vi "start.vi"(8 "error in (no error)":errorcluster, 11 "NetworkWinX32 in":refnum<class "NetworkWinX32.lvclass">) -> (0 "error out":errorcluster, 3 "NetworkWinX32 out":refnum<class "NetworkWinX32.lvclass">)   [LabVIEW 2011, in "Hardware.lvlib" / "HWControllers.lvlib" / "NetworkWinX32.lvclass"]
uses:
  NetworkWinX32.lvclass
  NetworkWinX32.lvclass/NetworkWinX32.ctl
  Channels/Camera/WinX32_SA/WinX32Camera.lvclass
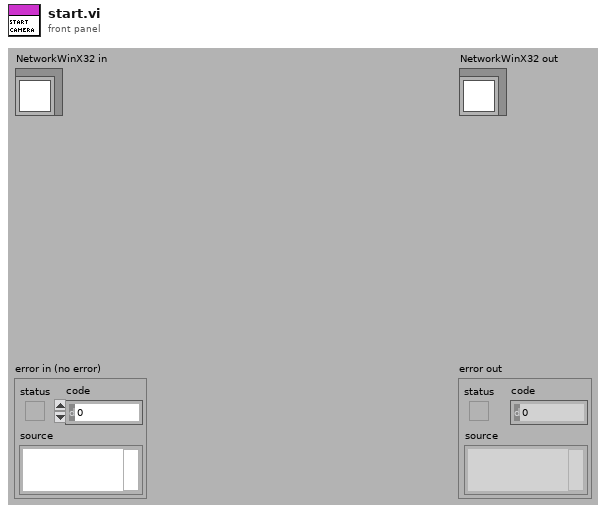
[diagram p1: front panel]
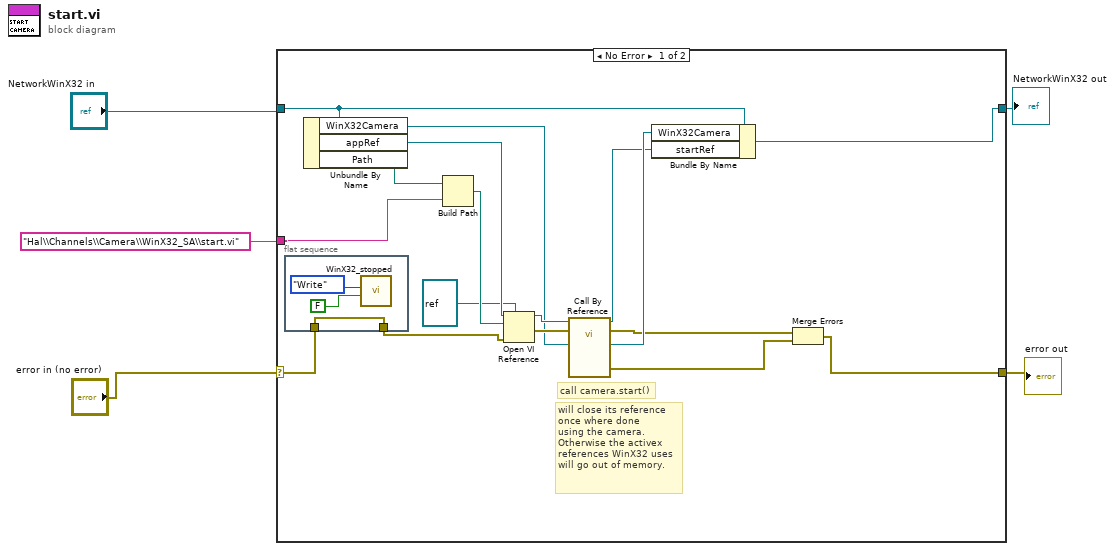
[diagram p0: block diagram]
diagram:
  n1 = case shown="No Error" "error in (no error)" {
    selector: "error in (no error)" -> [w9 w27]
    tunnel: [w11 w27] -> w2
    tunnel: [w10 w26] -> w3
    tunnel: "NetworkWinX32 in" -> [w14 w26]
    tunnel: "Hal\\Channels\\Camera\\WinX32_SA\\start.vi" ("viPath") -> [w21 _]
    frame No Error {
      # "will close its reference\nonce where done\nusing the camera.\nOtherwise the activex\nreferences WinX32 uses\nwill go out of memory."
      # "call camera.start()"
      n2 = flat-sequence {
        tunnel: w9 -> [w25]
        tunnel: [w25] -> w8
        frame #0 {
          n3 = call "WinX32_stopped.vi"("stop"=FALSE, "Action"=enum16{"Write", "Read"}."Write") -> ()  [unwired: 9 in, 1 out]
        }
      }
      n4 = Unbundle By Name(w14) -> ("WinX32Camera"=w15:refnum<class "WinX32Camera.lvclass">, "appRef"=w19:refnum<vi>, "Path"=w20:path)
      n5 = Build Path(base path=w20, name or relative path=w21) -> (appended path=w22:path)
      n6 = Open VI Reference(type specifier VI Refnum (for type only)=refnum<vi> refnum, application reference (local)=w19, vi path=w22, error in (no error)=w8) -> (vi reference=w17:refnum<vi>, error out=w16:errorcluster)  [unwired: 2 in]
      n7 = call-by-ref "?"(reference=w17, error in=w16, "WinX32Camera in"=w15) -> (reference out=w6:refnum<vi>, error out=w7:errorcluster, 0:"error out"=w12:errorcluster, "WinX32Camera out"=w13:refnum<class "WinX32Camera.lvclass">)  [unwired: 9 in]
      n8 = Bundle By Name(cluster=w14, "WinX32Camera"=w13, "startRef"=w6) -> (w10:refnum<class "NetworkWinX32.lvclass">)
      n9 = Merge Errors(w7, w12) -> (w11:errorcluster)
    }
    frame Error {
    }
  }
  "error out" <- w2
  "NetworkWinX32 out" <- w3
